vi "OpenMemoryMap.vi"(8 "error in (no error)":errorcluster) -> (0 "Error out":errorcluster)   [LabVIEW 2020]
doc: "Open a Memory Map Viewer\n\nAndre Koelewijn, 3 April 2021\nOpen a memory map visualization tool.\nThis will show the memory layers content"
uses:
  Gserver/controls/Typedef_Gviewer-Query.ctl
  Gserver/controls/Typedef_QueryType.ctl
  Gserver/Gserver.lvclass
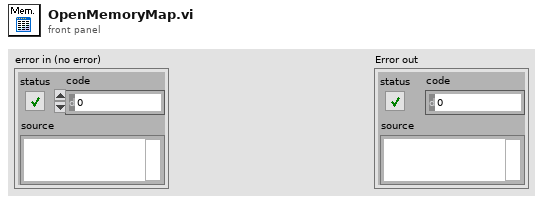
[diagram p1: front panel]
types:
  T1 = typedef "Sgraph_lib_V1.lvlib/Gserver.lvclass/Typedef_QueryType.ctl" = enum16{"Subscribe", "DataRequest", "RequestAllTags", "RequestIniPath", "FAMMstarted", "SetClientOptions", "GviewerUpdate", "OpenNewGraph", "CloseClient", "CloseAllClients", "Close Gserver", "OpenMemoryMap", "MeMapDataRequest", "MeMapDataResponse"}
  T2 = typedef "Sgraph_lib_V1.lvlib/Gserver.lvclass/Typedef_Gviewer-Query.ctl" = cluster{"Query_type":T1, "data":variant, "Source":string, "Time Stamp":timestamp}
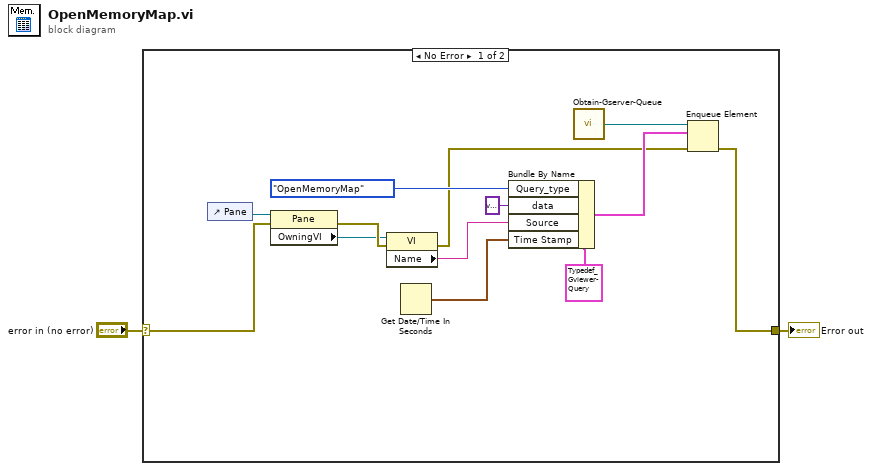
[diagram p0: block diagram]
diagram:
  n1 = case shown="No Error" "error in (no error)" {
    selector: "error in (no error)" -> [w9 w16]
    tunnel: [w6 w16] -> w1
    frame No Error {
      n2 = control-ref of="Pane"() -> (w11:refnum<vi>)
      n3 = property class="Pane"(reference=w11, error in=w9) -> (error out=w8:errorcluster, "OwningVI"=w4:refnum<vi>)  [unwired: 1 out]
      n4 = property class="VI"(reference=w4, error in=w8) -> (error out=w7:errorcluster, "Name"=w10:string)  [unwired: 1 out]
      n5 = Get Date/Time In Seconds() -> (seconds since 1Jan1904=w5:timestamp)
      n6 = Bundle By Name(cluster=T2 {"Query_type"=enum."Subscribe", "data"=variant, "Source"="", "Time Stamp"=timestamp(0 s since 1904-01-01)} ("element"), "Query_type"=Typedef_QueryType."OpenMemoryMap", "data"=variant, "Source"=w10, "Time Stamp"=w5) -> (w12:T2)
      n7 = call "Obtain-Gserver-Queue.vi"() -> ("Gserver Queue"=w15:refnum<queue>)  [unwired: 7 in]
      n8 = Enqueue Element(queue=w15, element=w12, error in (no error)=w7) -> (error out=w6:errorcluster)  [unwired: 1 in, 2 out]
    }
    frame Error {
    }
  }
  "Error out" <- w1
